vi "Last operation Record.vi"(8 "Error In":errorcluster, 9 "Operation":T1, 10 "FGV Choice":T2) -> (0 "Error Out":errorcluster, 2 "Last Operation":T1)   [LabVIEW 2019]
doc: "VI is used to set the value of last operation to allow the button to know what is next operation."
uses:
  FGV Selector.ctl
  Operation.ctl
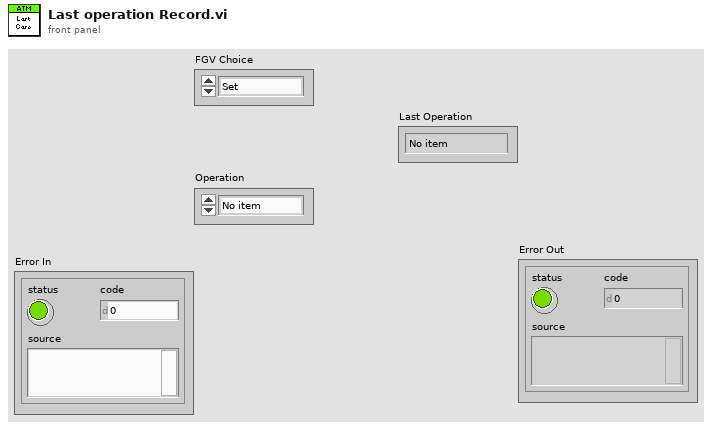
[diagram p1: front panel]
types:
  T1 = typedef "Operation.ctl" = enum16{"No item", "Card Inserted", "Deposit", "Withdrawn"}
  T2 = typedef "FGV Selector.ctl" = enum16{"Set", "Get"}
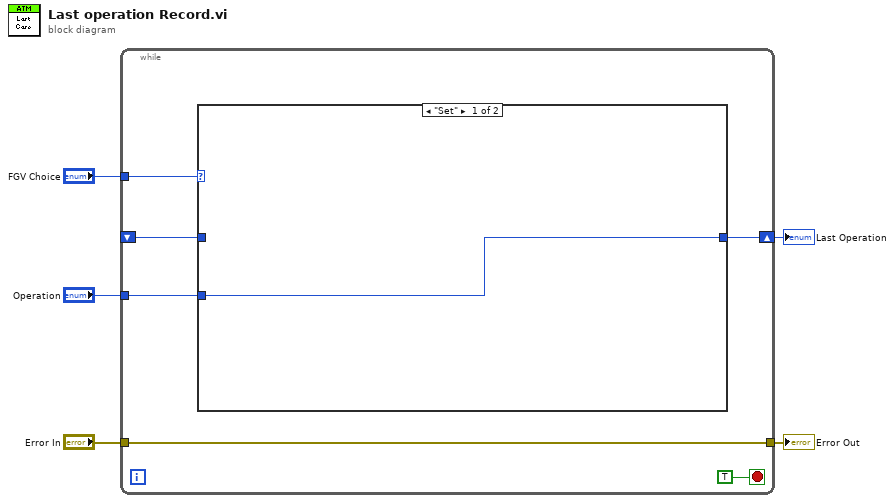
[diagram p0: block diagram]
diagram:
  n1 = while {
    tunnel: "FGV Choice" -> [w11]
    tunnel: "Operation" -> [w10]
    shift-right: [w9] -> w3
    shift-left: _ -> [w8]
    tunnel: "Error In" -> [w6]
    tunnel: [w6] -> w1
    stop <- TRUE stop-if-true
    n2 = case shown="\"Set\"" w11 {
      tunnel: w10 -> [w12 _]
      tunnel: [w12 w13] -> w9
      tunnel: w8 -> [_ w13]
      frame "Set" {
      }
      frame "Get", Default {
      }
    }
  }
  "Last Operation" <- w3
  "Error Out" <- w1
